vi "Joystick moved.vi"(9 "Threshold":dbl) -> (3 "Joystick moved":bool)   [LabVIEW 2010, in "Core SubVIs.lvlib"]
uses:
  Core SubVIs.lvlib
  Controls/TYPE - Analog Data Queue Method.ctl
  Instance           2 22Saved   Joystick moved .vi
  <vilib>/measure/madcrms.llb/Basic Averaged DC-RMS for 1 Chan.vi
  <vilib>/measure/NI_MAPro.lvlib
panel:
  in  "error in (no error)":errorcluster
  out "Up Joystick":bool caption="Up joystick"
  out "Down Joystick":bool caption="Down joystick"
  out "Left Joystick":bool caption="Left joystick"
  out "Right Joystick":bool caption="Right joystick"
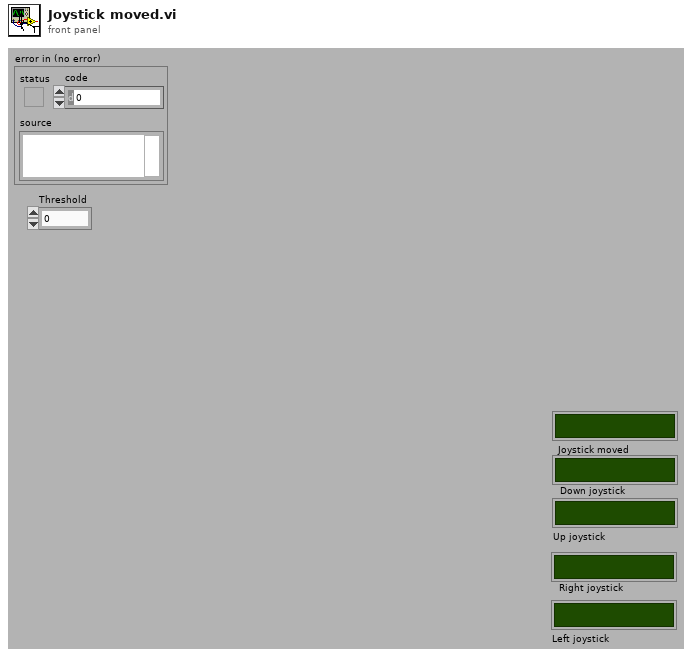
[diagram p1: front panel]
types:
  T1 = typedef "Core SubVIs.lvlib/TYPE - Analog Data Queue Method.ctl" = enum16{"Set Data Queue", "Preview Element", "Remove Element", "Get Data Queue", "Flush Data Queue"}
  T2 = typedef "Core SubVIs.lvlib/TYPE - Named Data Structures.ctl" = cluster{"Loop Name (DAQ Loop)":string, "queue out":refnum<queue>}
  T3 = typedef "Core SubVIs.lvlib/TYPE - Analog Data.ctl" = waveform(dbl)[]
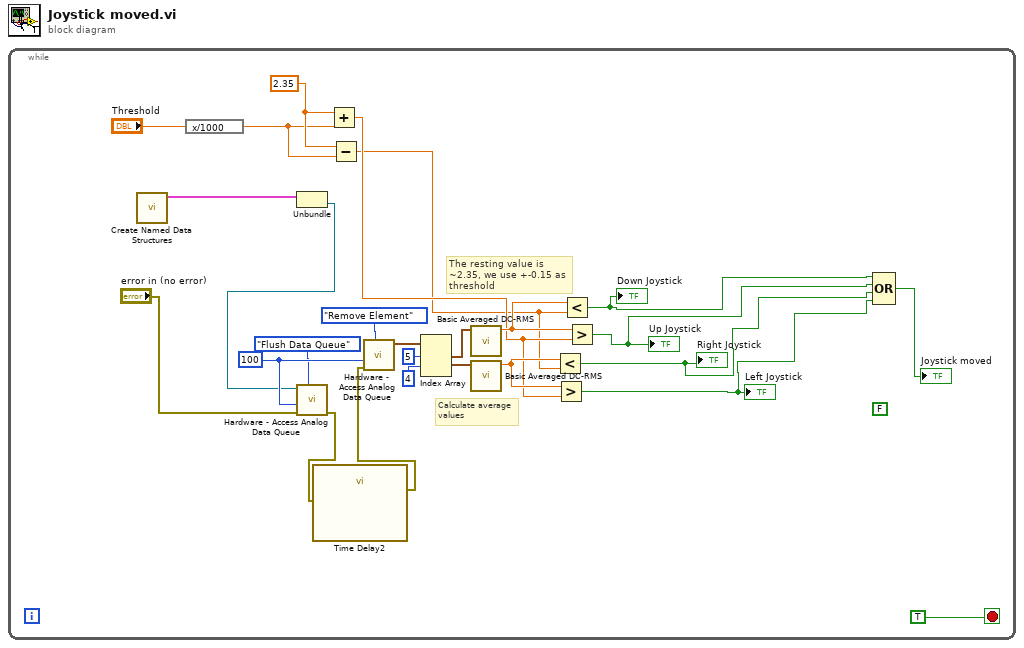
[diagram p0: block diagram]
diagram:
  n1 = while {
    stop <- TRUE stop-if-true
    w5 = 2.35
    (unwired) FALSE
    w14 = 100 ("timeout in ms (-1)")
    # "The resting value is ~2.35, we use +-0.15 as threshold"
    # "Calculate average\nvalues"
    n2 = call "Create Named Data Structures.vi"() -> ("Named Data Structures"=w12:T2)  [unwired: 10 in, 1 out]
    n3 = expression code="x/1000"("Threshold") -> (w1:dbl)
    n4 = Unbundle(w12) -> ("queue out"=w11:refnum<queue>)  [unwired: 1 out]
    n5 = call "Hardware - Access Analog Data Queue.vi"("Method"=TYPE_-_Analog_Data_Queue_Method."Flush Data Queue", "error in (no error)"="error in (no error)", "timeout in ms (-1)"=w14, "Analog Data Queue"=w11) -> ("error out"=w9:errorcluster)  [unwired: 4 in, 3 out]
    n6 = call "Time Delay2"("error in (no error)"=w9) -> ("error out"=w8:errorcluster)  [unwired: 10 in]
    n7 = Add(x=w5, y=w1) -> (x+y=w4:dbl)
    n8 = Subtract(x=w5, y=w1) -> (x-y=w3:dbl)
    n9 = call "Hardware - Access Analog Data Queue.vi"("Method"=TYPE_-_Analog_Data_Queue_Method."Remove Element", "error in (no error)"=w8, "timeout in ms (-1)"=w14) -> ("Analog Data"=w25:T3)  [unwired: 5 in, 3 out]
    n10 = Index Array(array=w25, index #1=5 ("index"), index #2=4 ("index")) -> (element #1=w24:waveform(dbl), element #2=w21:waveform(dbl))  [unwired: 1 in, 1 out]
    n11 = call-poly <vilib>:"Basic Averaged DC-RMS.vi"("signal in"=w24) -> ("DC value"=w23:dbl)  [unwired: 7 in, 3 out]
    n12 = call-poly <vilib>:"Basic Averaged DC-RMS.vi"("signal in"=w21) -> ("DC value"=w22:dbl)  [unwired: 7 in, 3 out]
    n13 = Less?(x=w22, y=w3) -> (x < y?=w17:bool)
    "Right Joystick" <- w17
    n14 = Greater?(x=w22, y=w4) -> (0:w16:bool)
    "Left Joystick" <- w16
    n15 = Less?(x=w23, y=w3) -> (x < y?=w19:bool)
    "Down Joystick" <- w19
    n16 = Greater?(x=w23, y=w4) -> (0:w18:bool)
    "Up Joystick" <- w18
    n17 = Compound Arithmetic op=OR(w19, w18, w17, w16) -> (→"Joystick moved":bool)
  }
